vi "FeedbackDecode_GenContMvnt.vi"(0 "Mode":enum16{"Initialize", "Reset", "Run"}(ring), 2 "LoopCount":dbl, 3 "LoopPeriod":u64=10 caption="Loop Period (ms)", 4 "Gain":dbl=1.0 min=-1.0 max=1.0, 5 "MvntClust":T1={"MvntMat"=[], "MvntName"="", "Tracking"=enum."False", "Radius"=0.15} {"Radius" min=0.0 max=1.0 step=0.01}) -> (6 "State":enum16{"Running", "Finished"}(ring)=enum."Finished", 7 "MaxTimes (ms)":T2, 8 "ContMvntVal":dbl[](array[numeric]))   [LabVIEW 2020]
uses:
  <vilib>/Analysis/NI_AALBase.lvlib
panel:
  out "ZeroMvntVal":dbl[](array[numeric])
  out "ContMvntArray":dbl[][](array[numeric])
  out "BaseCount":dbl
  # "Thumb"
  # "Index"
  # "Middle"
  # "Ring"
  # "Little"
  # "ThumbInt"
  # "IndexInt"
  # "RingInt"
  # "LittleInt"
  # "WristPitch"
  # "WristYaw"
  # "WristRoll"
  # "Amp"
  # "Del"
  # "Rise"
  # "Hold"
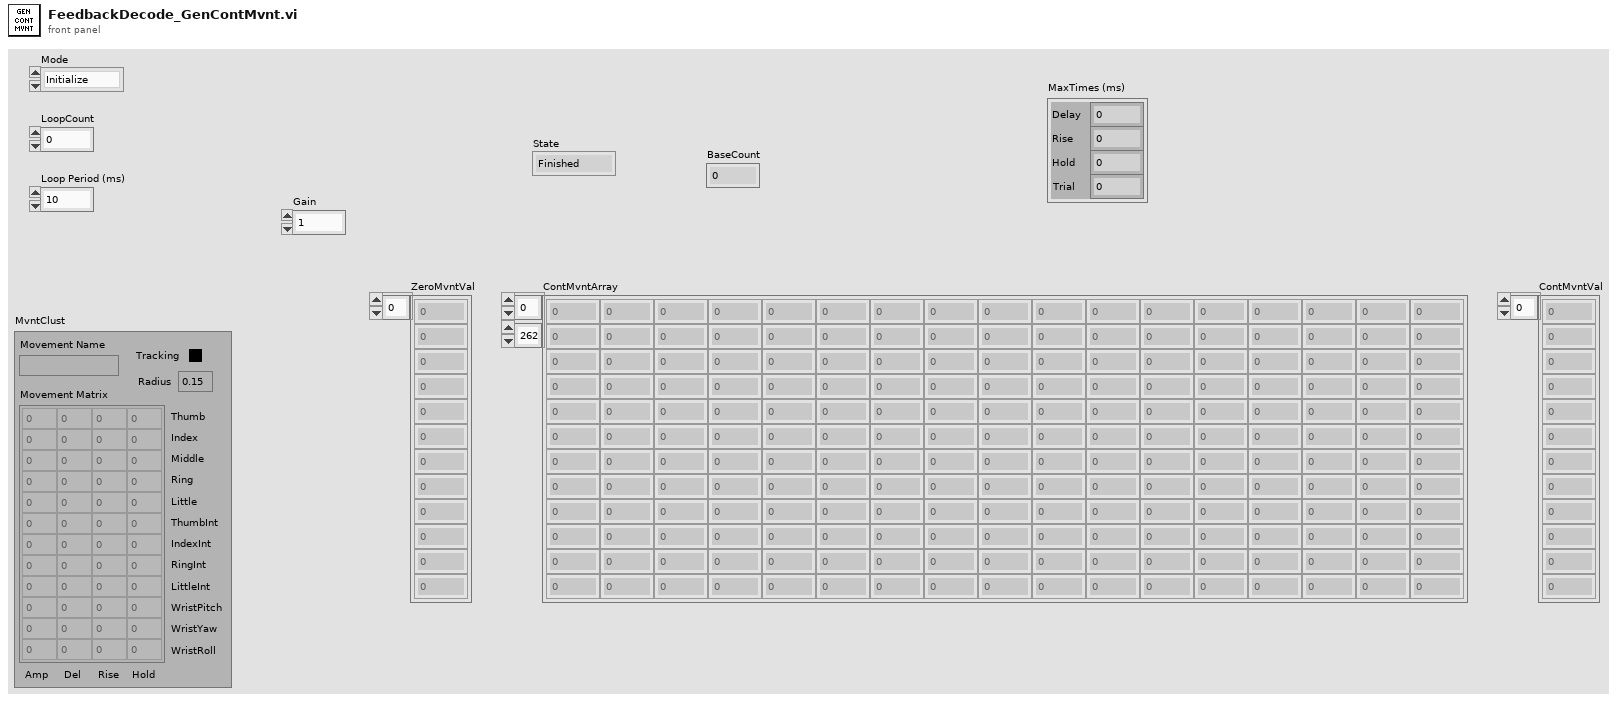
[diagram p1: front panel]
types:
  T1 = cluster{"MvntMat":dbl[][], "MvntName":string, "Tracking":enum8{"False", "True", "Mixed"}, "Radius":dbl}
  T2 = cluster{"Delay":dbl, "Rise":dbl, "Hold":dbl, "Trial":dbl}
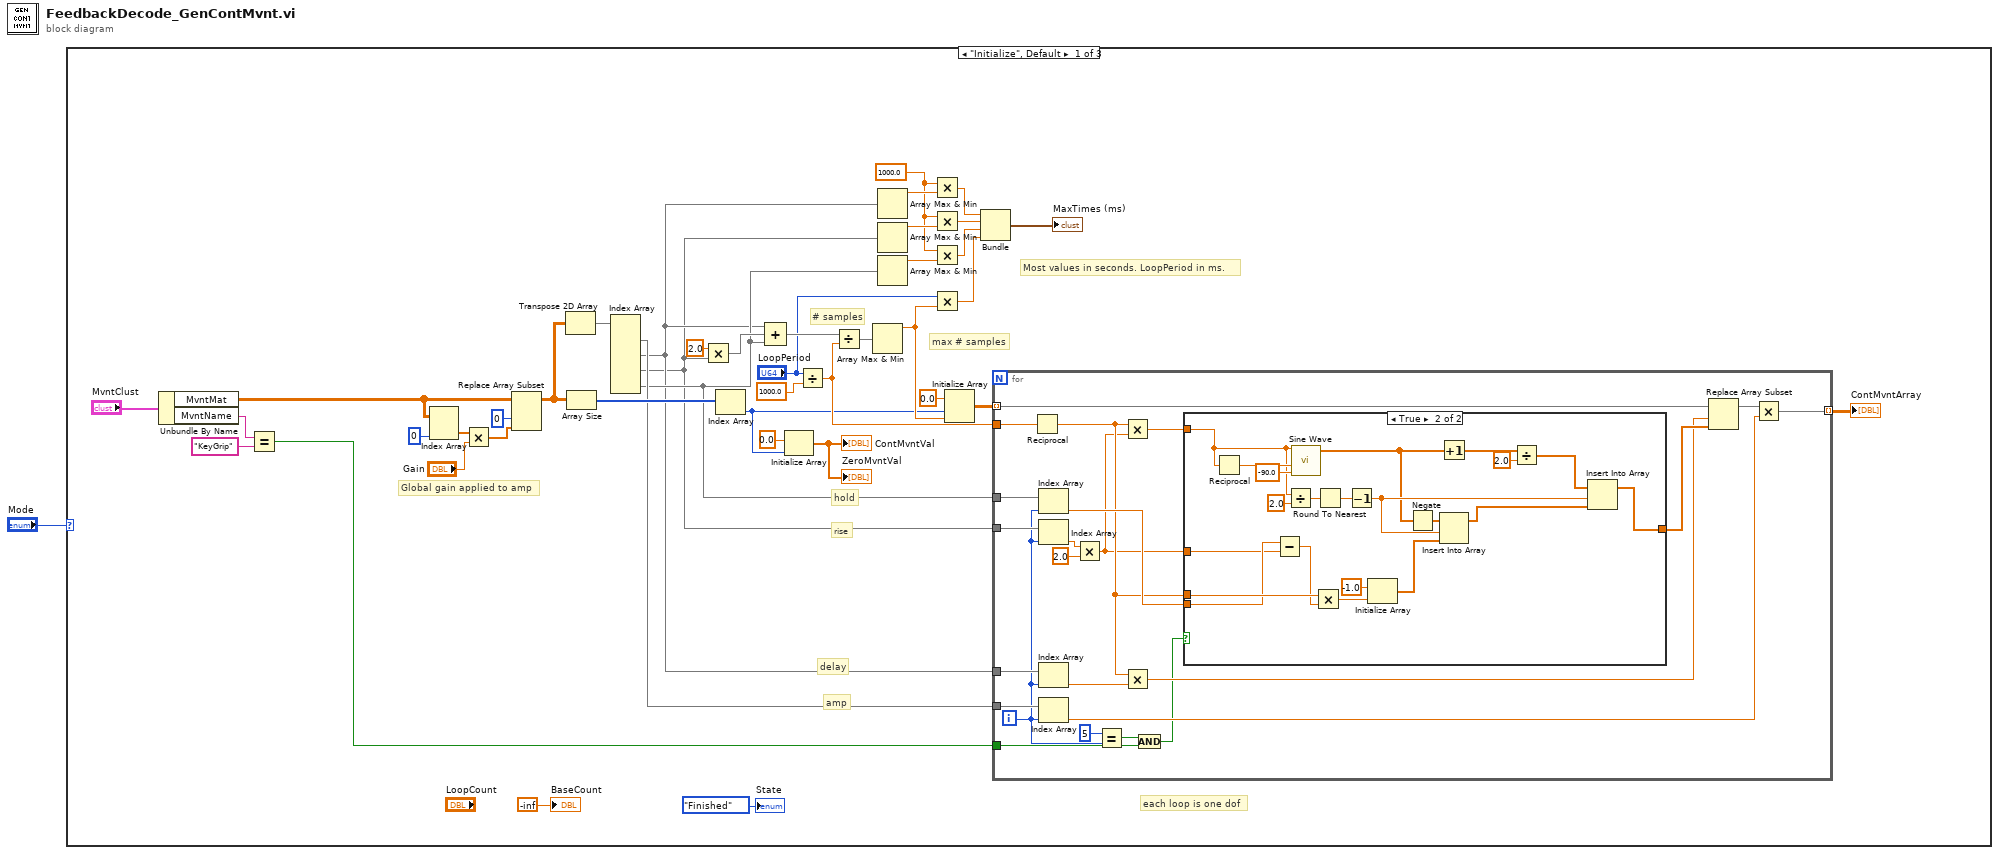
[diagram p0: block diagram]
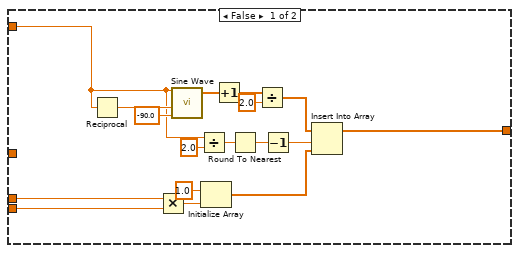
[diagram p2: hidden frame]
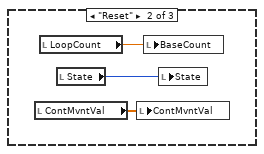
[diagram p3: hidden frame]
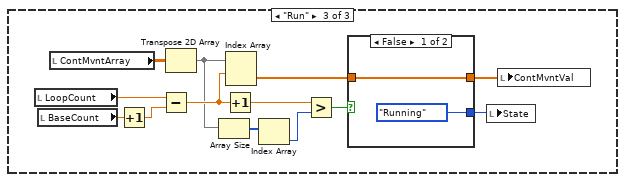
[diagram p4: hidden frame]
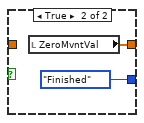
[diagram p5: hidden frame]
diagram:
  n1 = case shown="\"Initialize\", Default" "Mode" {
    frame "Initialize", Default {
      w12 = 1000.0 ("x")
      # "each loop is one dof"
      # "Global gain applied to amp"
      # "amp"
      # "max # samples"
      # "# samples"
      # "Most values in seconds. LoopPeriod in ms."
      # "hold"
      # "rise"
      # "delay"
      n2 = Unbundle By Name("MvntClust") -> ("MvntMat"=w4:dbl[][], "MvntName"=w39:string)
      n3 = Equal?(x=w39, y="KeyGrip") -> (x = y?=w3:bool)
      n4 = Index Array(array=w4, index (col)=0 ("disabled index (col)")) -> (element=w21:dbl[])  [unwired: 1 in]
      n5 = Multiply(x=w21, y="Gain") -> (x*y=w23:dbl[])
      n6 = Replace Array Subset(array=w4, new element=w23, index (col)=0 ("disabled index (col)")) -> (w19:dbl[][])  [unwired: 1 in]
      n7 = Transpose 2D Array(2D array=w19) -> (transposed array=w30:dbl[][])
      n8 = Array Size(array=w19) -> (size(s)=w29:i32[])
      n9 = Index Array(array=w30) -> (element #1=w25:dbl[], element #2=w16:dbl[], element #3=w15:dbl[], element #4=w18:dbl[])  [unwired: 8 in]
      n10 = Multiply(x=2.0, y=w15) -> (x*y=w32:dbl[])
      n11 = Index Array(array=w29) -> (element=w5:i32)  [unwired: 1 in]
      n12 = Compound Arithmetic op=ADD(w16, w32, w18) -> (w33:dbl[])
      n13 = Initialize Array(0.0 ("element"), w5) -> (→"ContMvntVal" →"ZeroMvntVal":dbl[])
      n14 = Divide(x="LoopPeriod", y=1000.0) -> (x/y=w26:dbl)
      n15 = Divide(x=w33, y=w26) -> (x/y=w35:dbl[])
      n16 = Array Max & Min(array=w35) -> (max value=w7:dbl)  [unwired: 3 out]
      n17 = Array Max & Min(array=w16) -> (max value=w13:dbl)  [unwired: 3 out]
      n18 = Array Max & Min(array=w15) -> (max value=w14:dbl)  [unwired: 3 out]
      n19 = Array Max & Min(array=w18) -> (max value=w17:dbl)  [unwired: 3 out]
      n20 = Multiply(x=w12, y=w13) -> (x*y=w11:dbl)
      n21 = Multiply(x=w12, y=w14) -> (x*y=w10:dbl)
      n22 = Multiply(x=w12, y=w17) -> (x*y=w9:dbl)
      n23 = Multiply(x="LoopPeriod", y=w7) -> (x*y=w6:dbl)
      n24 = Initialize Array(0.0, w5, w7) -> (w28:dbl[][])
      n25 = Bundle(w11, w10, w9, w6) -> (→"MaxTimes (ms)":cluster{dbl, dbl, dbl, dbl})  [unwired: 1 in]
      n26 = for {
        tunnel: w28 -> [w62] mode=indexing
        tunnel: w16 -> [w66]
        tunnel: w15 -> [w65]
        tunnel: w18 -> [w64]
        tunnel: w26 -> [w60]
        tunnel: [w52] -> w41 mode=indexing
        tunnel: w25 -> [w55]
        tunnel: w3 -> [w47]
        i -> [w50]
        n27 = Reciprocal(x=w60) -> (1/x=w57:dbl)
        n28 = Index Array(array=w64, index=w50) -> (element=w63:dbl)
        n29 = Index Array(array=w65, index=w50) -> (element=w59:dbl)
        n30 = Index Array(array=w66, index=w50) -> (element=w56:dbl)
        n31 = Index Array(array=w55, index=w50) -> (element=w53:dbl)
        n32 = Multiply(x=w59, y=2.0) -> (x*y=w44:dbl)
        n33 = Equal?(x=5, y=w50) -> (x = y?=w48:bool)
        n34 = Multiply(x=w57, y=w44) -> (x*y=w45:dbl)
        n35 = Multiply(x=w57, y=w56) -> (x*y=w51:dbl)
        n36 = And(x=w48, y=w47) -> (x .and. y?=w46:bool)
        n37 = case shown="True" w46 {
          tunnel: w63 -> [w73 w88]
          tunnel: [w72 w98] -> w61
          tunnel: w57 -> [w71 w97]
          tunnel: w45 -> [w67 w94]
          tunnel: w44 -> [_ w87]
          frame False {
            n38 = Reciprocal(x=w67) -> (1/x=w83:dbl)
            n39 = Multiply(x=w71, y=w73) -> (x*y=w69:dbl)
            n40 = call <vilib>:"Sine Wave.vi"("samples"=w67, "frequency"=w83, "phase in"=-90.0) -> ("sine wave"=w81:dbl[])  [unwired: 2 in, 2 out]
            n41 = Divide(x=w67, y=2.0) -> (x/y=w77:dbl)
            n42 = Initialize Array(1.0, w69) -> (w74:dbl[])
            n43 = Increment(x=w81) -> (x+1=w80:dbl[])
            n44 = Round To Nearest(number=w77) -> (nearest integer value=w76:dbl)
            n45 = Divide(x=w80, y=2.0) -> (x/y=w70:dbl[])
            n46 = Decrement(x=w76) -> (x-1=w75:dbl)
            n47 = Insert Into Array(array=w70, index=w75, new element=w74) -> (w72:dbl[])
          }
          frame True {
            n48 = Reciprocal(x=w94) -> (1/x=w104:dbl)
            n49 = Subtract(x=w88, y=w87) -> (x-y=w86:dbl)
            n50 = Divide(x=w94, y=2.0) -> (x/y=w100:dbl)
            n51 = call <vilib>:"Sine Wave.vi"("samples"=w94, "frequency"=w104, "phase in"=-90.0) -> ("sine wave"=w84:dbl[])  [unwired: 2 in, 2 out]
            n52 = Multiply(x=w97, y=w86) -> (x*y=w96:dbl)
            n53 = Round To Nearest(number=w100) -> (nearest integer value=w99:dbl)
            n54 = Decrement(x=w99) -> (x-1=w91:dbl)
            n55 = Initialize Array(-1.0, w96) -> (w90:dbl[])
            n56 = Negate(x=w84) -> (-x=w92:dbl[])
            n57 = Increment(x=w84) -> (x+1=w85:dbl[])
            n58 = Insert Into Array(array=w92, index=w91, new element=w90) -> (w89:dbl[])
            n59 = Divide(x=w85, y=2.0) -> (x/y=w93:dbl[])
            n60 = Insert Into Array(array=w93, index=w91, new element=w89) -> (w98:dbl[])
          }
        }
        n61 = Replace Array Subset(array=w62, new element=w61, index=w51) -> (w54:dbl[])
        n62 = Multiply(x=w54, y=w53) -> (x*y=w52:dbl[])
      }
      "ContMvntArray" <- w41
      "BaseCount" <- -inf
      "State" <- enum16{"Running", "Finished"}."Finished" ("State")
    }
    frame "Reset" {
      n63 = local read "ContMvntVal"() -> (w105:dbl[])
      n64 = local read "LoopCount"() -> (w107:dbl)
      n65 = local read "State"() -> (w106:enum16{"Running", "Finished"})
      n66 = local write "ContMvntVal"(w105) -> ()
      n67 = local write "BaseCount"(w107) -> ()
      n68 = local write "State"(w106) -> ()
    }
    frame "Run" {
      n69 = local read "LoopCount"() -> (w119:dbl)
      n70 = local read "BaseCount"() -> (w120:dbl)
      n71 = local read "ContMvntArray"() -> (w113:dbl[][])
      n72 = Increment(x=w120) -> (x+1=w118:dbl)
      n73 = Subtract(x=w119, y=w118) -> (x-y=w112:dbl)
      n74 = Transpose 2D Array(2D array=w113) -> (transposed array=w111:dbl[][])
      n75 = Array Size(array=w111) -> (size(s)=w110:i32[])
      n76 = Increment(x=w112) -> (x+1=w117:dbl)
      n77 = Index Array(array=w111, index (row)=w112) -> (element=w115:dbl[])  [unwired: 1 in]
      n78 = Index Array(array=w110) -> (element=w109:i32)  [unwired: 1 in]
      n79 = Greater?(x=w117, y=w109) -> (0:w116:bool)
      n80 = case shown="False" w116 {
        tunnel: w115 -> [w121 _]
        tunnel: [w121 w123] -> w108
        tunnel: [enum16{"Running", "Finished"}."Running" ("State") enum16{"Running", "Finished"}."Finished" ("State")] -> w114
        frame False {
        }
        frame True {
          n81 = local read "ZeroMvntVal"() -> (w123:dbl[])
        }
      }
      n82 = local write "State"(w114) -> ()
      n83 = local write "ContMvntVal"(w108) -> ()
    }
  }
